vi "Register gRPC Methods.vi"(8 "error in (no error)":errorcluster, 11 "Template Server in":refnum<class "HVC5.lvclass">) -> (0 "error out":errorcluster, 3 "Template Server out":refnum<class "HVC5.lvclass">)   [LabVIEW 2019, in "HVC5.lvlib" / "HVC5.lvclass"]
uses:
  HVC5.lvclass
  typeDefs/Server Internal UEs.ctl
  typeDefs/Server Internal Message.ctl
  typeDefs/Server gRPC UEs.ctl
  gRPC lvSupport/Server API/typeDefs/gRPCId Cluster.ctl
  gRPC lvSupport/Server API/typeDefs/grpcId.ctl
  HVC5.lvclass/HVC5.ctl
  gRPC lvSupport/gprc-lvsupport.lvlib
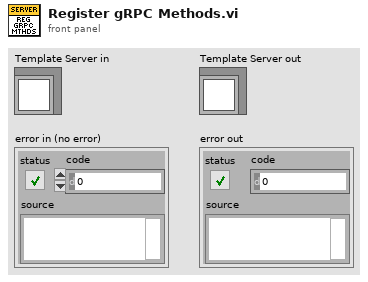
[diagram p1: front panel]
types:
  T1 = typedef "HVC5.lvlib/HVC5.lvclass/Server gRPC UEs.ctl" = cluster{"Invoke gRPC UE":refnum<user-event>, "Query gRPC UE":refnum<user-event>, "Register gRPC UE":refnum<user-event>, "OpenDMMSession gRPC UE":refnum<user-event>, "ConfigureDMM gRPC UE":refnum<user-event>, "PerformDMMVoltageMeasurement gRPC UE":refnum<user-event>, "CloseDMMSession gRPC UE":refnum<user-event>, "SelfCalibrateDMM gRPC UE":refnum<user-event>, "ResetDMM gRPC UE":refnum<user-event>, "OpenSMUSession gRPC UE":refnum<user-event>, "ConfigureSMU gRPC UE":refnum<user-event>, "EnableSMUOutput gRPC UE":refnum<user-event>, "DisableSMUOutput gRPC UE":refnum<user-event>, "PerformSMUCurrentMeasurement gRPC UE":refnum<user-event>, "CloseSMUSession gRPC UE":refnum<user-event>, "SelfCalibrateSMU gRPC UE":refnum<user-event>, "ResetSMU gRPC UE":refnum<user-event>, "OpenNI2576MUXSession gRPC UE":refnum<user-event>, "CloseNI2576MUXChannel gRPC UE":refnum<user-event>, "OpenNI2576MUXChannel gRPC UE":refnum<user-event>, "DisconnectAllNI2576MUXChannels gRPC UE":refnum<user-event>, "CloseNI2576MUXSession gRPC UE":refnum<user-event>, "ResetNI2576MUX gRPC UE":refnum<user-event>}
  T2 = typedef "HVC5.lvlib/HVC5.lvclass/Server Internal UEs.ctl" = cluster{"Invoke Internal UE":refnum<user-event>, "Query Internal UE":refnum<user-event>, "Register Internal UE":refnum<user-event>, "OpenDMMSession Internal UE":refnum<user-event>, "ConfigureDMM Internal UE":refnum<user-event>, "PerformDMMVoltageMeasurement Internal UE":refnum<user-event>, "CloseDMMSession Internal UE":refnum<user-event>, "SelfCalibrateDMM Internal UE":refnum<user-event>, "ResetDMM Internal UE":refnum<user-event>, "OpenSMUSession Internal UE":refnum<user-event>, "ConfigureSMU Internal UE":refnum<user-event>, "EnableSMUOutput Internal UE":refnum<user-event>, "DisableSMUOutput Internal UE":refnum<user-event>, "PerformSMUCurrentMeasurement Internal UE":refnum<user-event>, "CloseSMUSession Internal UE":refnum<user-event>, "SelfCalibrateSMU Internal UE":refnum<user-event>, "ResetSMU Internal UE":refnum<user-event>, "OpenNI2576MUXSession Internal UE":refnum<user-event>, "CloseNI2576MUXChannel Internal UE":refnum<user-event>, "OpenNI2576MUXChannel Internal UE":refnum<user-event>, "DisconnectAllNI2576MUXChannels Internal UE":refnum<user-event>, "CloseNI2576MUXSession Internal UE":refnum<user-event>, "ResetNI2576MUX Internal UE":refnum<user-event>}
  T3 = typedef "HVC5.lvlib/gprc-lvsupport.lvlib/grpcId.ctl" = u64
  T4 = typedef "HVC5.lvlib/HVC5.lvclass/Server Internal Message UE.ctl" = refnum<user-event>
  T5 = typedef "HVC5.lvlib/gprc-lvsupport.lvlib/gRPCId Cluster UE.ctl" = refnum<user-event>
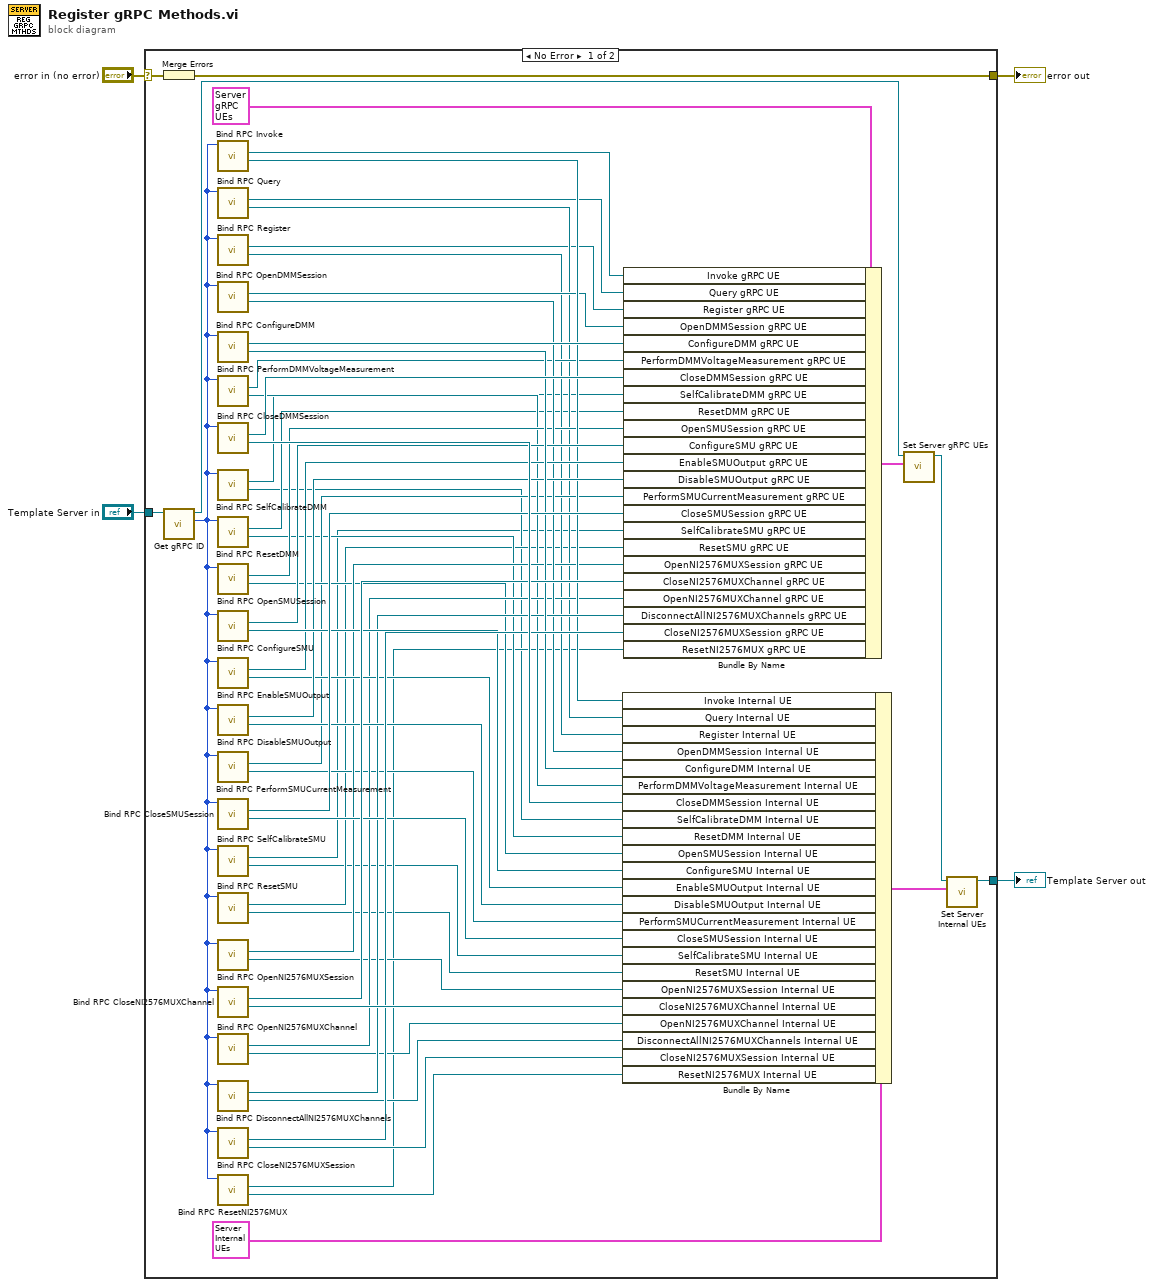
[diagram p0: block diagram]
diagram:
  n1 = case shown="No Error" "error in (no error)" {
    selector: "error in (no error)" -> [w52 w62]
    tunnel: "Template Server in" -> [w60 w63]
    tunnel: [w59 w62] -> w3
    tunnel: [w58 w63] -> w2
    frame No Error {
      n2 = Merge Errors(w52) -> (w59:errorcluster)
      n3 = call "Get gRPC ID.vi"("OOP Server in"=w60) -> ("gRPC ID"=w51:T3, "OOP Server out"=w61:refnum<class "HVC5.lvclass">)  [unwired: 9 in]
      n4 = call "Bind RPC Invoke.vi"("gRPCid server in"=w51) -> ("Invoke Internal UE"=w32:T4, "Invoke gRPC UE"=w31:T5)  [unwired: 7 in, 2 out]
      n5 = call "Bind RPC Query.vi"("gRPCid server in"=w51) -> ("Query Internal UE"=w18:T4, "Query gRPC UE"=w17:T5)  [unwired: 7 in, 2 out]
      n6 = call "Bind RPC Register.vi"("gRPCid server in"=w51) -> ("Register Internal UE"=w16:T4, "Register gRPC UE"=w15:T5)  [unwired: 7 in, 2 out]
      n7 = call "Bind RPC OpenDMMSession.vi"("gRPCid server in"=w51) -> ("OpenDMMSession Internal UE"=w30:T4, "OpenDMMSession gRPC UE"=w29:T5)  [unwired: 7 in, 2 out]
      n8 = call "Bind RPC ConfigureDMM.vi"("gRPCid server in"=w51) -> ("ConfigureDMM Internal UE"=w42:T4, "ConfigureDMM gRPC UE"=w41:T5)  [unwired: 7 in, 2 out]
      n9 = call "Bind RPC PerformDMMVoltageMeasurement.vi"("gRPCid server in"=w51) -> ("PerformDMMVoltageMeasurement Internal UE"=w22:T4, "PerformDMMVoltageMeasurement gRPC UE"=w21:T5)  [unwired: 7 in, 2 out]
      n10 = call "Bind RPC CloseDMMSession.vi"("gRPCid server in"=w51) -> ("CloseDMMSession Internal UE"=w50:T4, "CloseDMMSession gRPC UE"=w49:T5)  [unwired: 7 in, 2 out]
      n11 = call "Bind RPC SelfCalibrateDMM.vi"("gRPCid server in"=w51) -> ("SelfCalibrateDMM Internal UE"=w8:T4, "SelfCalibrateDMM gRPC UE"=w7:T5)  [unwired: 7 in, 2 out]
      n12 = call "Bind RPC ResetDMM.vi"("gRPCid server in"=w51) -> ("ResetDMM Internal UE"=w14:T4, "ResetDMM gRPC UE"=w13:T5)  [unwired: 7 in, 2 out]
      n13 = call "Bind RPC OpenSMUSession.vi"("gRPCid server in"=w51) -> ("OpenSMUSession Internal UE"=w24:T4, "OpenSMUSession gRPC UE"=w23:T5)  [unwired: 7 in, 2 out]
      n14 = call "Bind RPC ConfigureSMU.vi"("gRPCid server in"=w51) -> ("ConfigureSMU Internal UE"=w40:T4, "ConfigureSMU gRPC UE"=w39:T5)  [unwired: 7 in, 2 out]
      n15 = call "Bind RPC EnableSMUOutput.vi"("gRPCid server in"=w51) -> ("EnableSMUOutput Internal UE"=w34:T4, "EnableSMUOutput gRPC UE"=w33:T5)  [unwired: 7 in, 2 out]
      n16 = call "Bind RPC DisableSMUOutput.vi"("gRPCid server in"=w51) -> ("DisableSMUOutput Internal UE"=w38:T4, "DisableSMUOutput gRPC UE"=w37:T5)  [unwired: 7 in, 2 out]
      n17 = call "Bind RPC PerformSMUCurrentMeasurement.vi"("gRPCid server in"=w51) -> ("PerformSMUCurrentMeasurement Internal UE"=w20:T4, "PerformSMUCurrentMeasurement gRPC UE"=w19:T5)  [unwired: 7 in, 2 out]
      n18 = call "Bind RPC CloseSMUSession.vi"("gRPCid server in"=w51) -> ("CloseSMUSession Internal UE"=w44:T4, "CloseSMUSession gRPC UE"=w43:T5)  [unwired: 7 in, 2 out]
      n19 = call "Bind RPC SelfCalibrateSMU.vi"("gRPCid server in"=w51) -> ("SelfCalibrateSMU Internal UE"=w6:T4, "SelfCalibrateSMU gRPC UE"=w5:T5)  [unwired: 7 in, 2 out]
      n20 = call "Bind RPC ResetSMU.vi"("gRPCid server in"=w51) -> ("ResetSMU Internal UE"=w10:T4, "ResetSMU gRPC UE"=w9:T5)  [unwired: 7 in, 2 out]
      n21 = call "Bind RPC OpenNI2576MUXSession.vi"("gRPCid server in"=w51) -> ("OpenNI2576MUXSession Internal UE"=w26:T4, "OpenNI2576MUXSession gRPC UE"=w25:T5)  [unwired: 7 in, 2 out]
      n22 = call "Bind RPC CloseNI2576MUXChannel.vi"("gRPCid server in"=w51) -> ("CloseNI2576MUXChannel Internal UE"=w48:T4, "CloseNI2576MUXChannel gRPC UE"=w47:T5)  [unwired: 7 in, 2 out]
      n23 = call "Bind RPC OpenNI2576MUXChannel.vi"("gRPCid server in"=w51) -> ("OpenNI2576MUXChannel Internal UE"=w28:T4, "OpenNI2576MUXChannel gRPC UE"=w27:T5)  [unwired: 7 in, 2 out]
      n24 = call "Bind RPC DisconnectAllNI2576MUXChannels.vi"("gRPCid server in"=w51) -> ("DisconnectAllNI2576MUXChannels Internal UE"=w36:T4, "DisconnectAllNI2576MUXChannels gRPC UE"=w35:T5)  [unwired: 7 in, 2 out]
      n25 = call "Bind RPC CloseNI2576MUXSession.vi"("gRPCid server in"=w51) -> ("CloseNI2576MUXSession Internal UE"=w46:T4, "CloseNI2576MUXSession gRPC UE"=w45:T5)  [unwired: 7 in, 2 out]
      n26 = call "Bind RPC ResetNI2576MUX.vi"("gRPCid server in"=w51) -> ("ResetNI2576MUX Internal UE"=w12:T4, "ResetNI2576MUX gRPC UE"=w11:T5)  [unwired: 7 in, 2 out]
      n27 = Bundle By Name ("Bundle Internal UEs")(cluster=T2 {"Invoke Internal UE"=refnum, "Query Internal UE"=refnum, "Register Internal UE"=refnum, "OpenDMMSession Internal UE"=refnum, "ConfigureDMM Internal UE"=refnum, "PerformDMMVoltageMeasurement Internal UE"=refnum, "CloseDMMSession Internal UE"=refnum, "SelfCalibrateDMM Internal UE"=refnum, "ResetDMM Internal UE"=refnum, "OpenSMUSession Internal UE"=refnum, "ConfigureSMU Internal UE"=refnum, "EnableSMUOutput Internal UE"=refnum, "DisableSMUOutput Internal UE"=refnum, "PerformSMUCurrentMeasurement Internal UE"=refnum, "CloseSMUSession Internal UE"=refnum, "SelfCalibrateSMU Internal UE"=refnum, "ResetSMU Internal UE"=refnum, "OpenNI2576MUXSession Internal UE"=refnum, "CloseNI2576MUXChannel Internal UE"=refnum, "OpenNI2576MUXChannel Internal UE"=refnum, "DisconnectAllNI2576MUXChannels Internal UE"=refnum, "CloseNI2576MUXSession Internal UE"=refnum, "ResetNI2576MUX Internal UE"=refnum} ("Server Internal UEs"), "Invoke Internal UE"=w32, "Query Internal UE"=w18, "Register Internal UE"=w16, "OpenDMMSession Internal UE"=w30, "ConfigureDMM Internal UE"=w42, "PerformDMMVoltageMeasurement Internal UE"=w22, "CloseDMMSession Internal UE"=w50, "SelfCalibrateDMM Internal UE"=w8, "ResetDMM Internal UE"=w14, "OpenSMUSession Internal UE"=w24, "ConfigureSMU Internal UE"=w40, "EnableSMUOutput Internal UE"=w34, "DisableSMUOutput Internal UE"=w38, "PerformSMUCurrentMeasurement Internal UE"=w20, "CloseSMUSession Internal UE"=w44, "SelfCalibrateSMU Internal UE"=w6, "ResetSMU Internal UE"=w10, "OpenNI2576MUXSession Internal UE"=w26, "CloseNI2576MUXChannel Internal UE"=w48, "OpenNI2576MUXChannel Internal UE"=w28, "DisconnectAllNI2576MUXChannels Internal UE"=w36, "CloseNI2576MUXSession Internal UE"=w46, "ResetNI2576MUX Internal UE"=w12) -> (w57:T2)
      n28 = Bundle By Name ("Bundle gRPC UEs")(cluster=T1 {"Invoke gRPC UE"=refnum, "Query gRPC UE"=refnum, "Register gRPC UE"=refnum, "OpenDMMSession gRPC UE"=refnum, "ConfigureDMM gRPC UE"=refnum, "PerformDMMVoltageMeasurement gRPC UE"=refnum, "CloseDMMSession gRPC UE"=refnum, "SelfCalibrateDMM gRPC UE"=refnum, "ResetDMM gRPC UE"=refnum, "OpenSMUSession gRPC UE"=refnum, "ConfigureSMU gRPC UE"=refnum, "EnableSMUOutput gRPC UE"=refnum, "DisableSMUOutput gRPC UE"=refnum, "PerformSMUCurrentMeasurement gRPC UE"=refnum, "CloseSMUSession gRPC UE"=refnum, "SelfCalibrateSMU gRPC UE"=refnum, "ResetSMU gRPC UE"=refnum, "OpenNI2576MUXSession gRPC UE"=refnum, "CloseNI2576MUXChannel gRPC UE"=refnum, "OpenNI2576MUXChannel gRPC UE"=refnum, "DisconnectAllNI2576MUXChannels gRPC UE"=refnum, "CloseNI2576MUXSession gRPC UE"=refnum, "ResetNI2576MUX gRPC UE"=refnum} ("gRPC Server Method Events"), "Invoke gRPC UE"=w31, "Query gRPC UE"=w17, "Register gRPC UE"=w15, "OpenDMMSession gRPC UE"=w29, "ConfigureDMM gRPC UE"=w41, "PerformDMMVoltageMeasurement gRPC UE"=w21, "CloseDMMSession gRPC UE"=w49, "SelfCalibrateDMM gRPC UE"=w7, "ResetDMM gRPC UE"=w13, "OpenSMUSession gRPC UE"=w23, "ConfigureSMU gRPC UE"=w39, "EnableSMUOutput gRPC UE"=w33, "DisableSMUOutput gRPC UE"=w37, "PerformSMUCurrentMeasurement gRPC UE"=w19, "CloseSMUSession gRPC UE"=w43, "SelfCalibrateSMU gRPC UE"=w5, "ResetSMU gRPC UE"=w9, "OpenNI2576MUXSession gRPC UE"=w25, "CloseNI2576MUXChannel gRPC UE"=w47, "OpenNI2576MUXChannel gRPC UE"=w27, "DisconnectAllNI2576MUXChannels gRPC UE"=w35, "CloseNI2576MUXSession gRPC UE"=w45, "ResetNI2576MUX gRPC UE"=w11) -> (w54:T1)
      n29 = call "Set Server gRPC UEs.vi"("Server gRPC UEs"=w54, "OOP Server in"=w61) -> ("OOP Server out"=w55:refnum<class "HVC5.lvclass">)  [unwired: 9 in]
      n30 = call "Set Server Internal UEs.vi"("Server Internal UEs"=w57, "OOP Server in"=w55) -> ("OOP Server out"=w58:refnum<class "HVC5.lvclass">)  [unwired: 9 in]
    }
    frame Error {
    }
  }
  "error out" <- w3
  "Template Server out" <- w2
